vi "Test DAQmx tags.vi"() -> ()   [LabVIEW 2020]
uses:
  <vilib>/JDP Science/JSONtext/JSONtext.lvlib
panel:
  out "x = y?":bool
  out "<JSON>":string
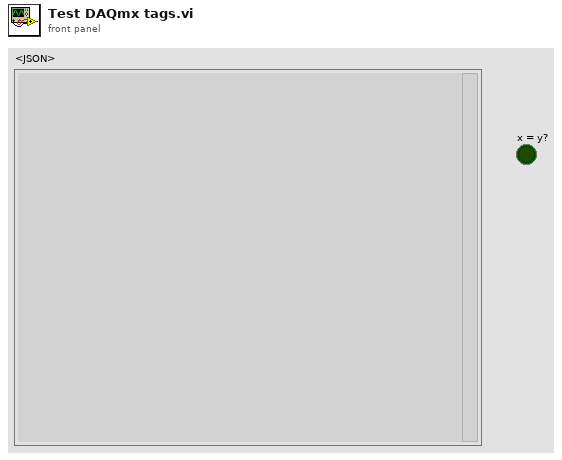
[diagram p1: front panel]
types:
  T1 = cluster{"DAQmx Task Name":refnum<k21>, "DAQmx Global Channel":refnum<k21>, "DAQmx Scale Name":tag, "DAQmx Terminal":tag, "DAQmx Device Name":tag, "DAQmx Physical Channel":tag}
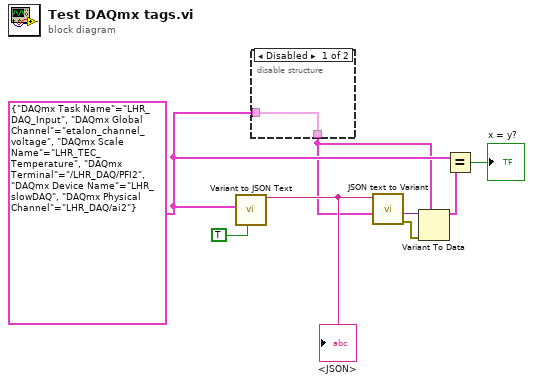
[diagram p0: block diagram]
diagram:
  w7 = T1 {"DAQmx Task Name"="LHR_DAQ_Input", "DAQmx Global Channel"="etalon_channel_voltage", "DAQmx Scale Name"="LHR_TEC_Temperature", "DAQmx Terminal"="/LHR_DAQ/PFI2", "DAQmx Device Name"="LHR_slowDAQ", "DAQmx Physical Channel"="LHR_DAQ/ai2"}
  n1 = call <vilib>:"Variant to JSON Text.vi"("Pretty Print?"=TRUE, "Variant"=w7) -> ("<JSON>"=w8:string)  [unwired: 7 in, 2 out]
  "<JSON>" <- w8
  n2 = disable-structure shown="Disabled" {
    disable-tunnel: w7 -> [w9 _]
    disable-tunnel: [w9 _] -> w3
    frame Disabled {
    }
    frame Enabled {
    }
  }
  n3 = call <vilib>:"JSON text to Variant.vi"("Data Type"=w3, "JSON"=w8) -> ("error out"=w5:errorcluster, "Variant out"=w4:variant)  [unwired: 8 in]
  n4 = Variant To Data(error in=w5, type=w3, Variant=w4) -> (data=w2:T1)  [unwired: 1 out]
  n5 = Equal?(x=w7, y=w2) -> (x = y?=→"x = y?":bool)
